vi "PWM (Single Output).vi"(5 "Clock Select":u8, 7 "Counter Control":u8 format="%08b", 10 "Output Compare Value":u16, 11 "Max Counter Value":u16) -> (2 "Output":bool, 3 "Counter Value":u16)   [LabVIEW 2016]
doc: "This VI generates one PWM signal using a single-clock source."
panel:
  # "This VI generates one PWM signal using a single-clock source."
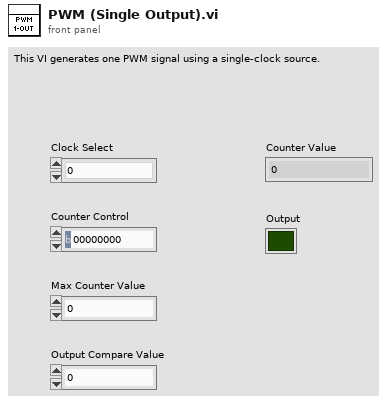
[diagram p1: front panel]
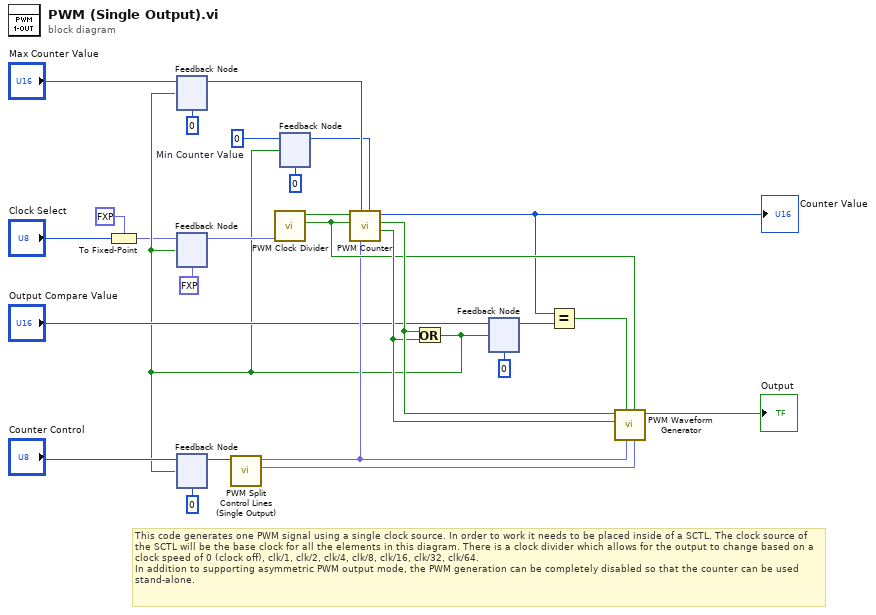
[diagram p0: block diagram]
diagram:
  w14 = u16 0  # Min Counter Value
  # "This code generates one PWM signal using a single clock source. In order to work it needs to be placed inside of a SCTL. The clock source of the SCTL will be the base clock for all the elements in this diagram. There is a clock divider which allows for the output to change based on a clock speed of 0 (clock off), clk/1, clk/2, clk/4, clk/8, clk/16, clk/32, clk/64. \nIn addition to supporting asymmetric PWM output mode, the PWM generation can be completely disabled so that the counter can be used stand-alone."
  n1 = To Fixed-Point(fixed-point type=fxp<+,3,3> 0.0 ("Clock Select"), number="Clock Select") -> (fixed-point=w2:fxp<+,3,3>)
  n2 = feedback #1(u16 0 ("Output Compare Value")) -> (w15:u16)
  n3 = feedback #2(fxp<+,3,3> 0.0 ("Clock Select")) -> (w9:fxp<+,3,3>)
  n4 = feedback #3(u8 0 ("Counter Control")) -> (w6:u8)
  n5 = call "PWM Split Control Lines (Single Output).vi"("Counter Control"=w6) -> ("Compare Output Mode"=w21:fxp<+,2,2>, "Waveform Generation Mode"=w22:fxp<+,2,2>)  [unwired: 9 in]
  n6 = call "PWM Clock Divider.vi"("Clock Select"=w9) -> ("Enable"=w23:bool, "Reset"=w27:bool)  [unwired: 9 in]
  n7 = feedback #4(u16 0 ("Output Compare Value")) -> (w13:u16)
  n8 = call "PWM Counter.vi"("Min Counter Value"=w13, "Waveform Generation Mode"=w22, "Max Counter Value"=w15, "Enable"=w23, "Reset"=w27) -> ("Counter is Min?"=w24:bool, "Counter is Max?"=w25:bool, "Counter Value"=w20:u16)  [unwired: 4 in]
  "Counter Value" <- w20
  n9 = Or(x=w25, y=w24) -> (x .or. y?=w4:bool)
  n10 = feedback-in #1("Max Counter Value", w4) -> ()
  n11 = feedback-in #2(w2, w4) -> ()
  n12 = feedback-in #3("Counter Control", w4) -> ()
  n13 = feedback-in #4(w14, w4) -> ()
  n14 = feedback-in #5("Output Compare Value", w4) -> ()
  n15 = feedback #5(u16 0 ("Output Compare Value")) -> (w17:u16)
  n16 = Equal?(x=w20, y=w17) -> (x = y?=w19:bool)
  n17 = call "PWM Waveform Generator.vi"("Compare Output Mode"=w21, "Enable In"=w23, "Waveform Generation Mode"=w22, "Counter is Output Compare?"=w19, "Counter is Min?"=w24, "Counter is Max?"=w25) -> ("Output"=→"Output":bool)  [unwired: 5 in]
